vi "Lid Unlock Retries.vi"(0 "GEA2 Reference In":refnum<k24>, 7 "Standalone?":bool, 11 "Error In":errorcluster) -> (4 "GEA2 Reference Out":refnum<k24>, 6 "Pass/Fail?":bool, 8 "Report Text":string="Upper Limit, Lower Limit, and Results Arrays must all be equal size and not be zero. If results array is all zeros, device may have shutdown.", 10 "Results":dbl[][](array[numeric])=[[0.991, 0.02, 2.505, 0.02, 2.5060000000000002, 0.02, 2.505, 0.02, 32.514, 0.021, 2.513, 0.021, 2.505, 0.02, 2.505, 0.02, 56.294000000000004]], 15 "Error Out":errorcluster)   [LabVIEW 2016, in "Centauro.lvlib"]
doc: "This vi confirms timing of lid lock algorithm"
uses:
  Projects/Centauro.lvlib
  Q:/Common/DLLs/GEA3/GeaCommunication.dll
  Common/DLLs/GEA3/GeaCommunication.dll
  Common/LabVIEW GEA2 Toolkit/LabVIEW_GEA2_Toolkit.lvlibp/type defs/Source_Destination.ctl
  Common/LabVIEW GEA2 Toolkit/LabVIEW_GEA2_Toolkit.lvlibp/type defs/ERD Write Data In.ctl
  Common/LabVIEW GEA2 Toolkit/LabVIEW_GEA2_Toolkit.lvlibp/type defs/Data Type.ctl
  <vilib>/DAQmx/read.llb/DAQmx Read (Digital Wfm 1Chan NSamp).vi
  <vilib>/DAQmx/create/channels.llb/DAQmx Create Channel (DI-Digital Input).vi
  <vilib>/DAQmx/configure/timing.llb/DAQmx Timing (Sample Clock).vi
  <vilib>/DAQmx/miscellaneous.llb/DAQmx Fill In Error Info.vi
  Common/LabVIEW GEA2 Toolkit/LabVIEW_GEA2_Toolkit.lvlibp
panel:
  in  "Lower Limits":dbl[][](array[numeric])=[[3.0, 0.016, 1.0, 0.016, 1.0, 0.016, 1.0, 0.016, 1.0, 0.016, 235.0, 0.016, 1.0, 0.016, 1.0, 0.016, 1.0, 0.016, 225.0]]
  in  "Upper Limits":dbl[][](array[numeric])=[[7.0, 0.034, 3.0, 0.034, 3.0, 0.034, 3.0, 0.034, 3.0, 0.034, 265.0, 0.034, 3.0, 0.034, 3.0, 0.034, 3.0, 0.034, 60.0]]
  out "Digital Waveform Graph":digitalwaveform(graph)={"t0"=timestamp(3515843915.9003177 s since 1904-01-01), "dt"=0.001, "Y"={"transitions"=[], "data"=array105000x1[105000 elements]}, "attributes"=variant("NI_ChannelName"=variant(string "9401_1/port0/line2"), "NI_LineNames"=variant(string "9401_1/port0/line2"))}
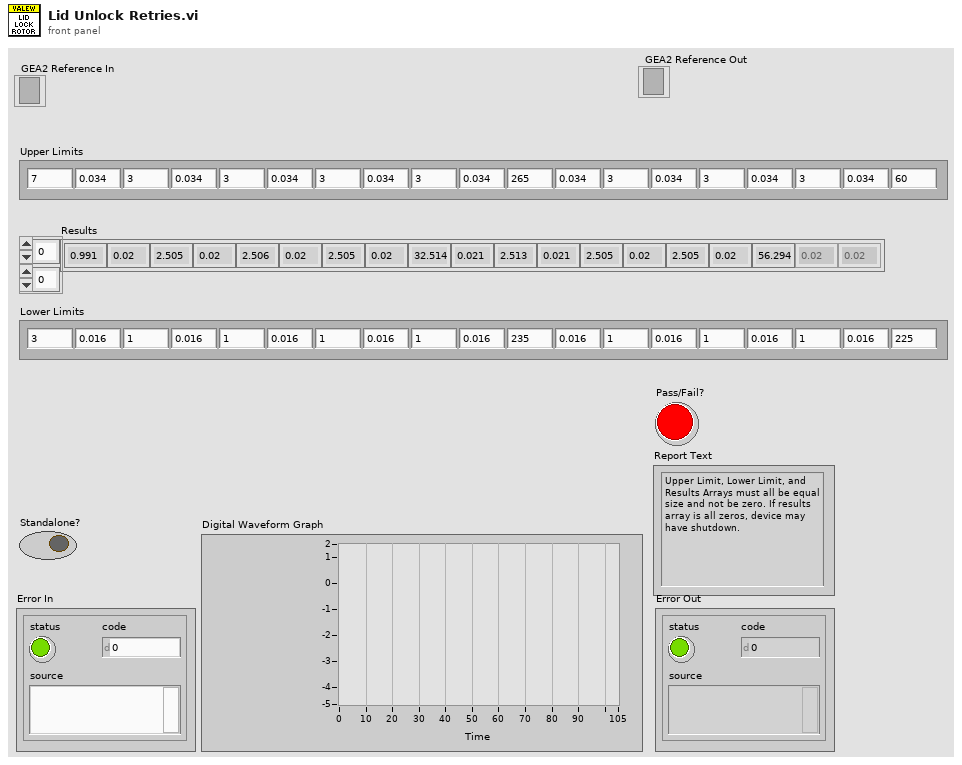
[diagram p1: front panel]
types:
  T1 = typedef "LabVIEW_GEA2_Toolkit.lvlibp/ERD Write Data In.ctl" = cluster{"ERD Number":u16, "Data Type":T2, "Data":string}
  T2 = typedef "LabVIEW_GEA2_Toolkit.lvlibp/Data Type.ctl" = enum16{"string", "boolean", "uint8_t", "uint16_t", "uint32_t", "uint64_t", "int8_t", "int16_t", "int32_t", "int64_t"}
  T3 = typedef "LabVIEW_GEA2_Toolkit.lvlibp/Source_Destination.ctl" = cluster{"Source":u8, "Destination":u8}
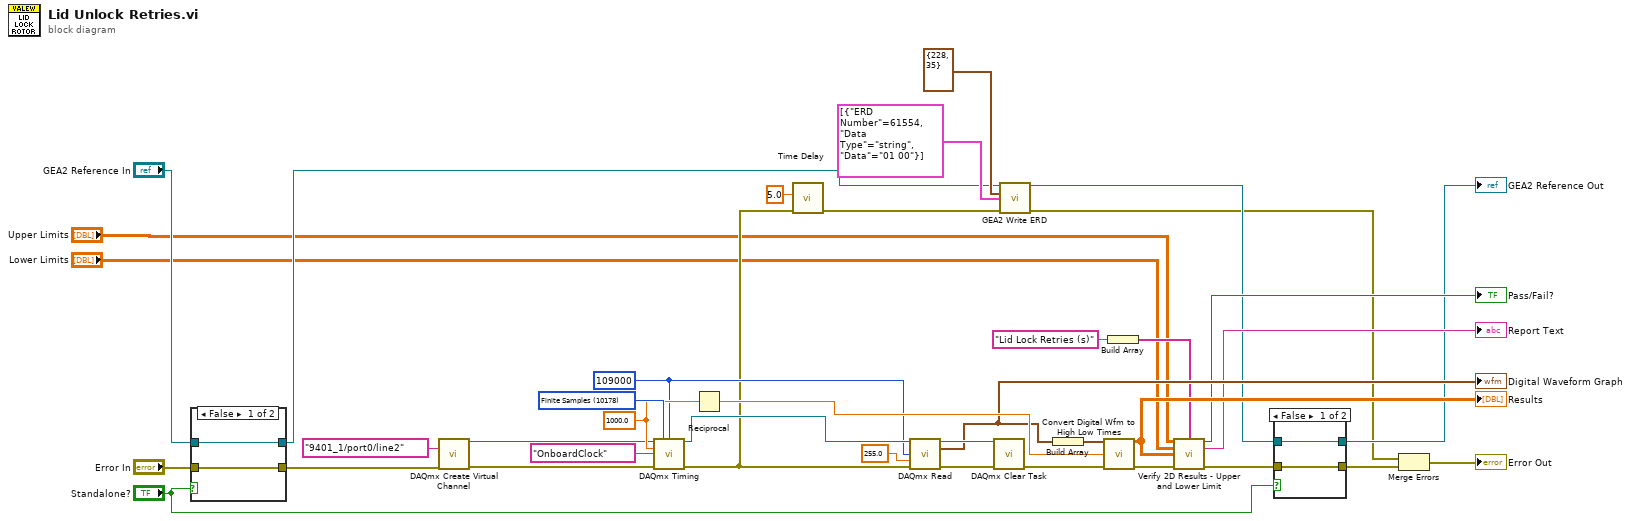
[diagram p0: block diagram]
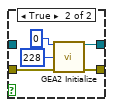
[diagram p2: hidden frame]
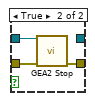
[diagram p3: hidden frame]
diagram:
  w38 = 10178 items=["Finite Samples"=10178, "Continuous Samples"=10123, "Hardware Timed Single Point"=12522] ("sample mode")
  w25 = 109000 ("samples per channel")
  w35 = 1000.0 ("rate")
  n1 = case shown="False" "Standalone?" {
    tunnel: "Error In" -> [w40 w46]
    tunnel: [w40 w45] -> w9
    tunnel: "GEA2 Reference In" -> [w41 _]
    tunnel: [w41 w44] -> w3
    frame False {
    }
    frame True {
      n2 = call "GEA2 Initialize.vi"("Board Index"=0, "Source Address"=u8 228, "error in"=w46) -> ("GEA2 Reference Out"=w44:refnum<k24>, "error out"=w45:errorcluster)  [unwired: 10 in, 1 out]
    }
  }
  n3 = call-poly <vilib>:"DAQmx Create Virtual Channel.vi"("lines"=tag "9401_1/port0/line2", "error in"=w9) -> ("task out"=w27:refnum<k21>, "error out"=w26:errorcluster)  [unwired: 12 in]
  n4 = call-poly <vilib>:"DAQmx Timing.vi"("task/channels in"=w27, "sample mode"=w38, "samples per channel"=w25, "rate"=w35, "source"=tag "OnboardClock", "error in"=w26) -> ("task out"=w28:refnum<k21>, "error out"=w6:errorcluster)  [unwired: 8 in]
  n5 = Reciprocal(x=w35) -> (1/x=w34:dbl)
  n6 = call "Time Delay"("error in (no error)"=w6, "Delay Time (s)"=5.0) -> ("error out"=w5:errorcluster)  [unwired: 9 in]
  n7 = call-poly <vilib>:"DAQmx Read.vi"("task/channels in"=w28, "number of samples per channel"=w25, "timeout"=255.0, "error in"=w6) -> ("task out"=w32:refnum<k21>, "data"=w30:digitalwaveform, "error out"=w33:errorcluster)  [unwired: 9 in]
  "Digital Waveform Graph" <- w30
  n8 = call <vilib>:"DAQmx Clear Task.vi"("task in"=w32, "error in"=w33) -> ("error out"=w31:errorcluster)  [unwired: 13 in]
  n9 = call "GEA2 Write ERD.vi"("GEA2 Reference In"=w3, "GEA Inputs"=T3 {"Source"=228, "Destination"=35}, "Write ERD List"=T1[] [{"ERD Number"=61554, "Data Type"=enum."string", "Data"="01 00"}], "Error In"=w5) -> ("GEA2 Reference Out"=w14:refnum<k24>, "Error Out"=w12:errorcluster)  [unwired: 9 in, 1 out]
  n10 = Build Array(w30) -> (w36:digitalwaveform[])
  n11 = call "Convert Digital Wfm to High Low Times.vi"("Digital Waveform In"=w36, "Dt"=w34, "Error In"=w31) -> ("HL Raw Output"=w24:dbl[][], "Error Out"=w23:errorcluster)  [unwired: 11 in]
  "Results" <- w24
  n12 = Build Array("Lid Lock Retries (s)" ("String")) -> (w21:string[])
  n13 = call "Verify 2D Results - Upper and Lower Limit.vi"("Upper Limits"="Upper Limits", "Array of Names"=w21, "Lower Limits"="Lower Limits", "Results"=w24, "Error In"=w23) -> ("Pass/Fail?"=→"Pass/Fail?":bool, "Report Text"=→"Report Text":string, "Error Out"=w16:errorcluster)  [unwired: 7 in, 1 out]
  n14 = case shown="False" "Standalone?" {
    tunnel: w16 -> [w48 w51]
    tunnel: [w48 w50] -> w13
    tunnel: [w47 _] -> w15
    tunnel: w14 -> [w47 w49]
    frame False {
    }
    frame True {
      n15 = call "GEA2 Stop.vi"("GEA2 Reference In"=w49, "Error In"=w51) -> ("Error Out"=w50:errorcluster)  [unwired: 13 in]
    }
  }
  "GEA2 Reference Out" <- w15
  n16 = Merge Errors(w12, w13) -> (→"Error Out":errorcluster)
